vi "Set NamedBundler Input Count.vi"(8 "error in (no error)":errorcluster, 10 "Numeric":i32, 11 "NamedBundler in":refnum<vi>) -> (0 "error out":errorcluster, 3 "NamedBundler out":refnum<vi>)   [LabVIEW 2019, in "gRPC Scripting Tools.lvlib"]
uses:
  gRPC Scripting Tools.lvlib
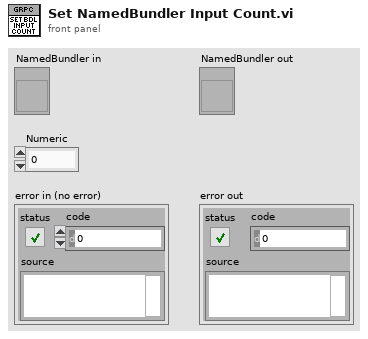
[diagram p1: front panel]
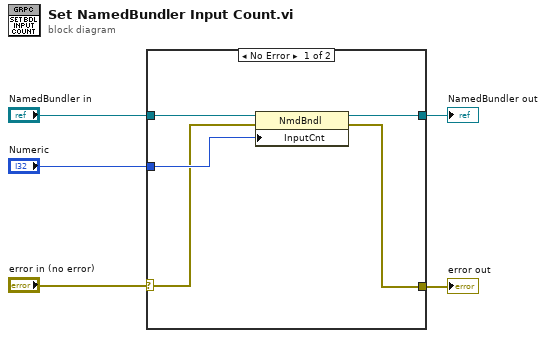
[diagram p0: block diagram]
diagram:
  n1 = case shown="No Error" "error in (no error)" {
    selector: "error in (no error)" -> [w6 w12]
    tunnel: [w10 w12] -> w5
    tunnel: [w9 w11] -> w4
    tunnel: "NamedBundler in" -> [w8 w11]
    tunnel: "Numeric" -> [w7 _]
    frame No Error {
      n2 = property class="NmdBndl"(reference=w8, error in=w6, "InputCnt"=w7) -> (reference out=w9:refnum<vi>, error out=w10:errorcluster)
    }
    frame Error {
    }
  }
  "error out" <- w5
  "NamedBundler out" <- w4
